vi "Main.vi"(8 "error in":errorcluster, 11 "Front Panel Emulator in":refnum<class "Front Panel Emulator.lvclass">) -> (0 "error out":errorcluster, 3 "Front Panel Emulator out":refnum<class "Front Panel Emulator.lvclass">)   [LabVIEW 2017, in "Front Panel Emulator.lvclass"]
doc: "The <b>Queued Message Handler</b> of the Worker that owns this VI."
uses:
  Front Panel Emulator.lvclass
  C:/Program Files (x86)/National Instruments/LabVIEW 2017/vi.lib/addons/_Workers/Library/Classes/Worker/Worker.lvclass
  Initialization Data.ctl
  Response Cases.ctl
  <vilib>/addons/_Workers/Library/Case Label.ctl
  Front Panel Emulator.lvclass/Front Panel Emulator.ctl
  rql_Position Changed.ctl
  rsp_Set Position.ctl
  <vilib>/addons/_Workers/Library/Classes/Message/Priority.ctl
  rql_Update LCD.ctl
  rqp_Update Temperature.ctl
  rqp_Update Humidity.ctl
  <vilib>/addons/_Workers/Library/Classes/Message Queue/Message Queue.lvclass
  <vilib>/addons/_Workers/Library/Workers.lvlib
  <vilib>/addons/_Workers/Library/Classes/Message/Message.lvclass
panel:
  in  "Position":dbl(knob) min=0.0 max=180.0 scale=0.0..180.0
  out "LCD":string
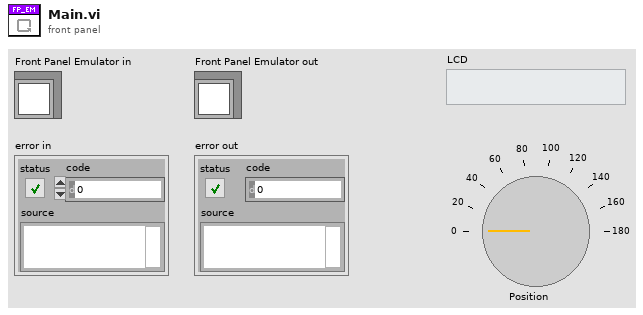
[diagram p1: front panel]
types:
  T1 = typedef "Front Panel Emulator.lvclass/Initialization Data.ctl" = cluster{"Response Cases":T2}
  T2 = typedef "Front Panel Emulator.lvclass/Response Cases.ctl" = cluster{"Set Position":T3}
  T3 = typedef "Workers.lvlib/Case Label.ctl" = string
  T4 = typedef "Front Panel Emulator.lvclass/rsp_Set Position.ctl" = cluster{"Position":dbl}
  T5 = typedef "Front Panel Emulator.lvclass/rql_Position Changed.ctl" = cluster{"Placeholder":string}
  T6 = typedef "Front Panel Emulator.lvclass/rql_Update LCD.ctl" = cluster{"Placeholder":string}
  T7 = typedef "Front Panel Emulator.lvclass/rqp_Update Temperature.ctl" = cluster{"Temperature":dbl}
  T8 = typedef "Front Panel Emulator.lvclass/rqp_Update Humidity.ctl" = cluster{"Humidity":dbl}
  T9 = typedef "Workers.lvlib/Message.lvclass/Priority.ctl" = enum16{"Low", "Normal", "High"}
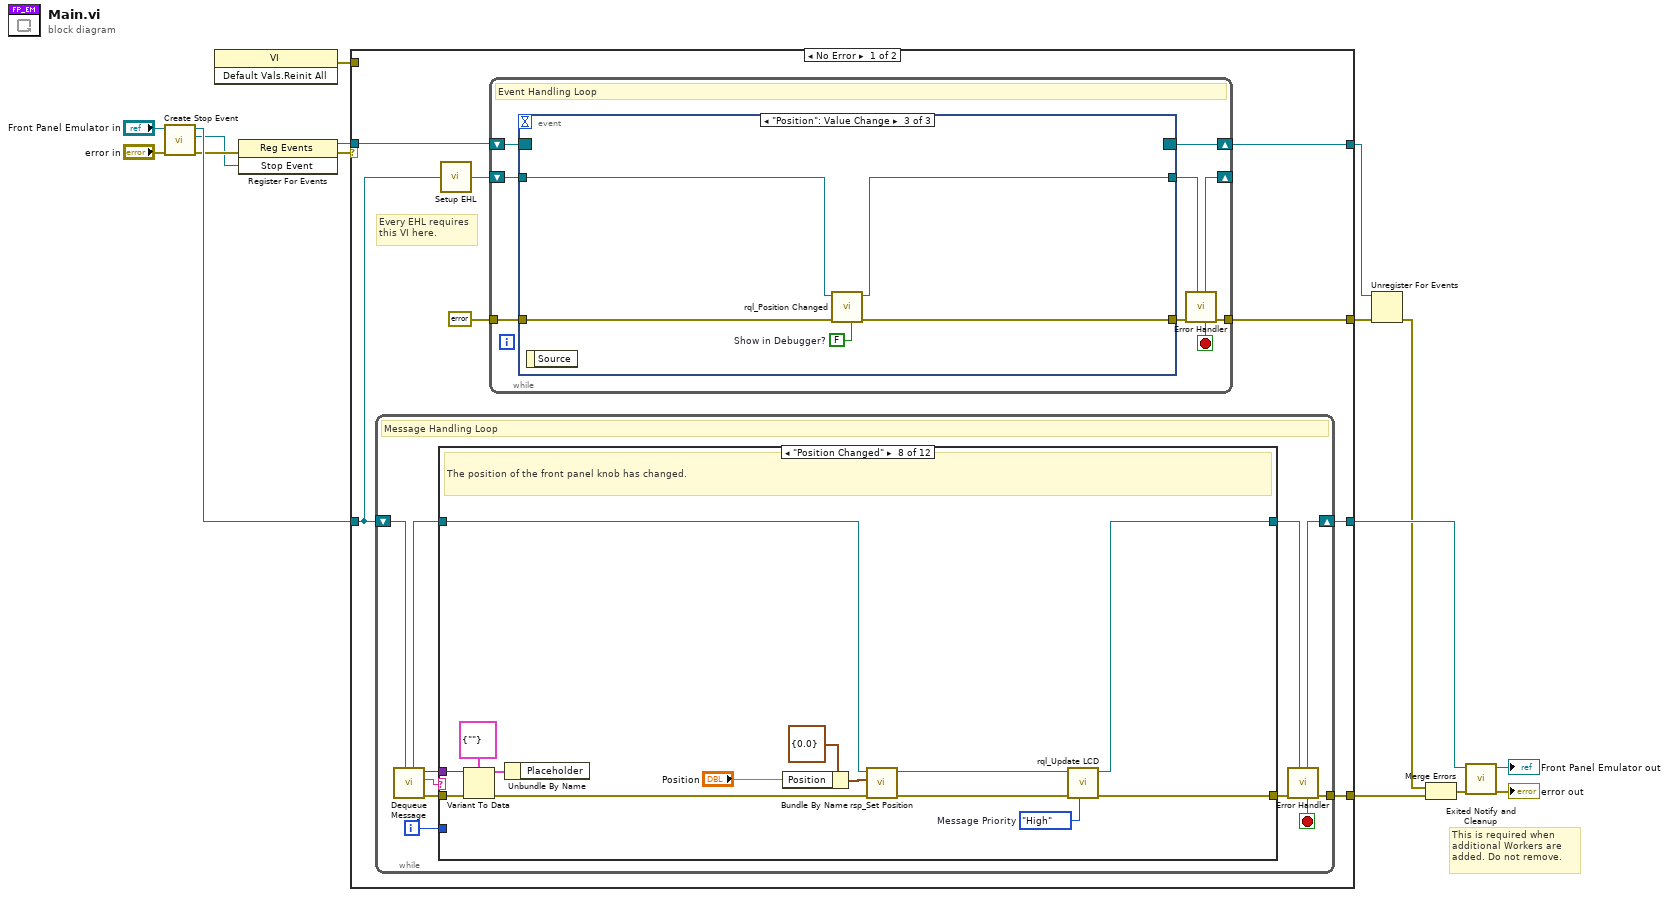
[diagram p0: block diagram]
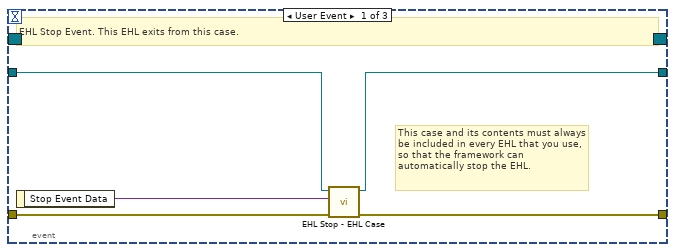
[diagram p2: hidden frame]
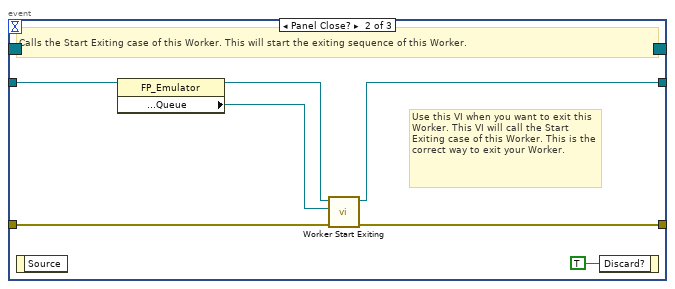
[diagram p3: hidden frame]
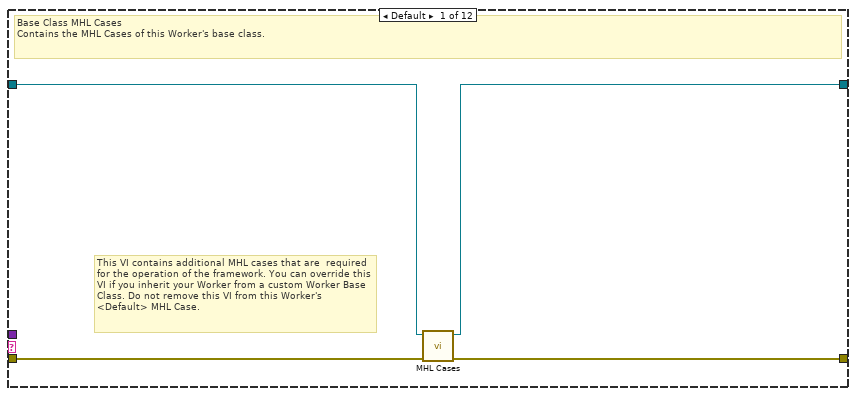
[diagram p4: hidden frame]
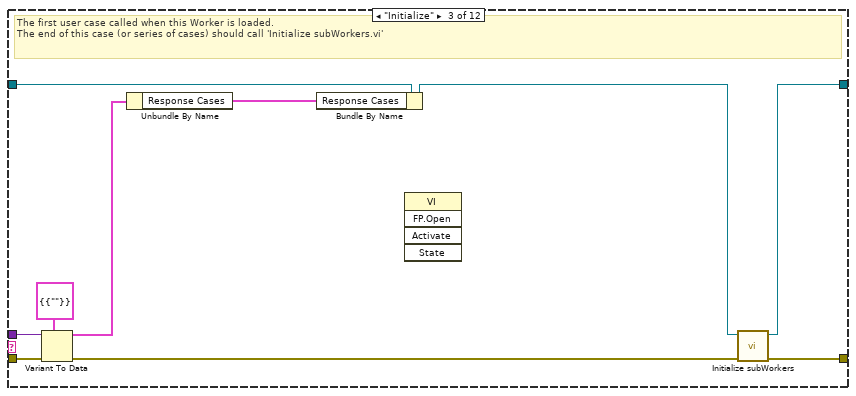
[diagram p6: hidden frame]
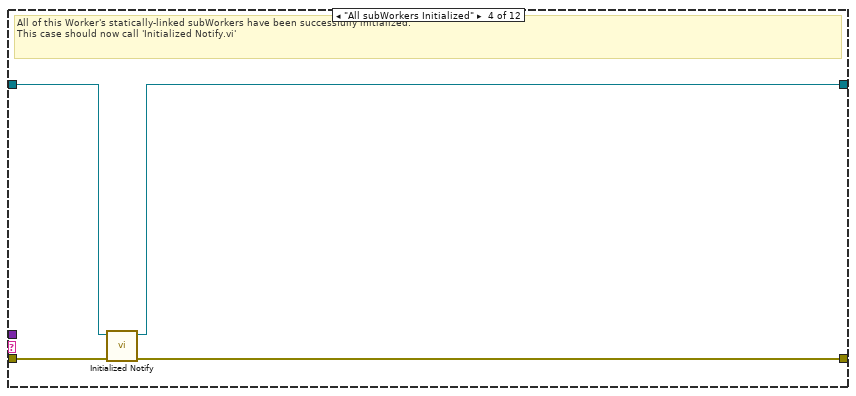
[diagram p7: hidden frame]
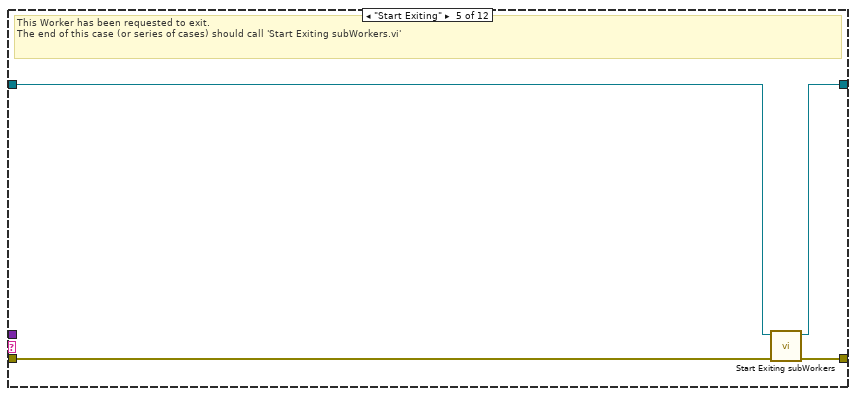
[diagram p8: hidden frame]
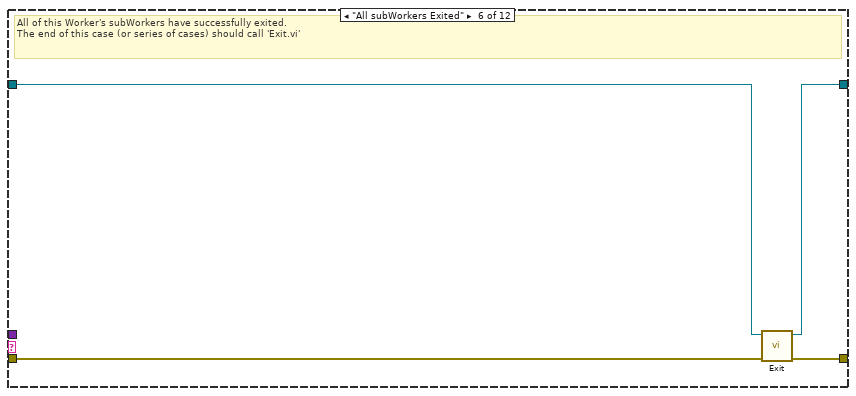
[diagram p9: hidden frame]
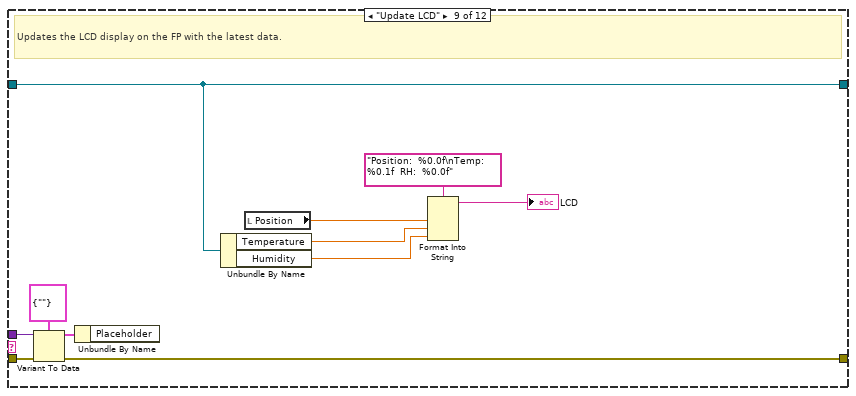
[diagram p11: hidden frame]
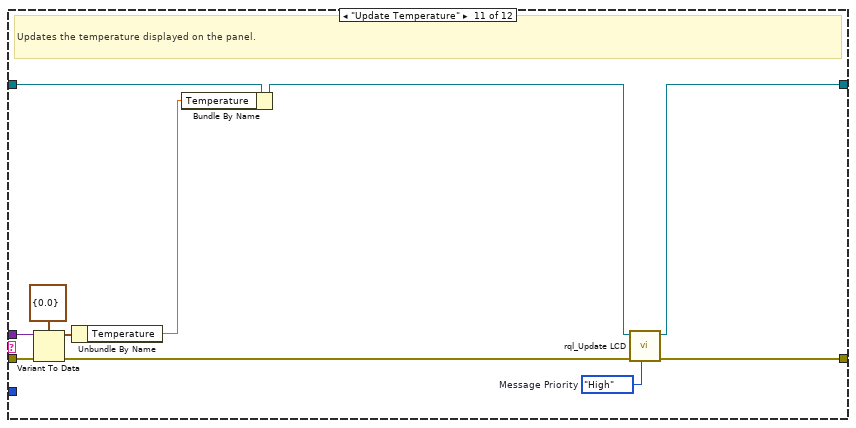
[diagram p13: hidden frame]
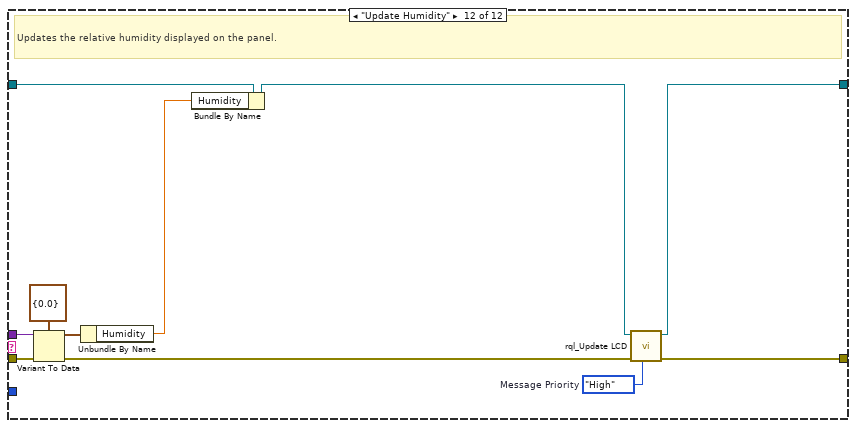
[diagram p14: hidden frame]
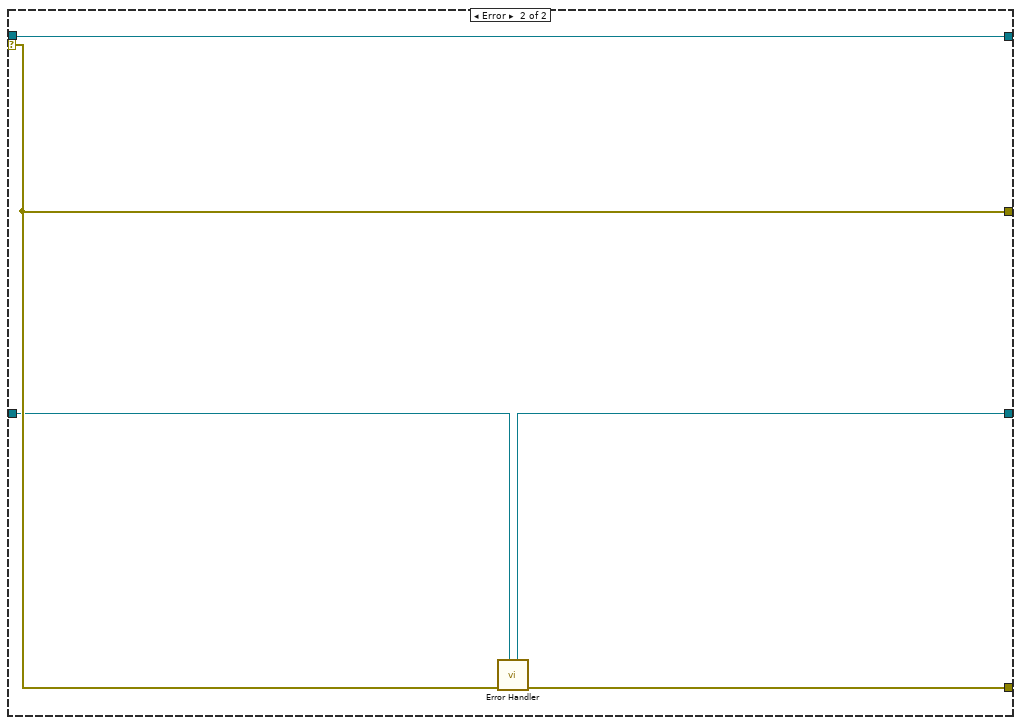
[diagram p15: hidden frame]
diagram:
  # "This is required when additional Workers are added. Do not remove."
  n1 = call-dynamic "Create Stop Event.vi"("error in"="error in", "Worker"="Front Panel Emulator in") -> ("error out"=w9:errorcluster, "Stop Event"=w8:refnum<user-event>, "Worker out"=w11:refnum<class "Front Panel Emulator.lvclass">)  [unwired: 7 in]
  n2 = invoke class="VI" method="Default Vals.Reinit All"() -> (error out=w1:errorcluster)  [unwired: 3 in, 2 out]
  n3 = register-events(error in=w9, w8) -> (reference out=w5:refnum<event-registration>, error out=w10:errorcluster)  [unwired: 1 in]
  n4 = case shown="No Error" w10 {
    tunnel: w11 -> [w22 w143]
    tunnel: [w24 w144] -> w15
    tunnel: [w23 w142] -> w16
    selector: w10 -> [_ w145]
    tunnel: w5 -> [w19 w141]
    tunnel: [w18 w141] -> w4
    tunnel: [w17 w145] -> w3
    tunnel: w1 -> [_ _]
    frame No Error {
      # "Every EHL requires\nthis VI here."
      n5 = while {
        shift-right: [w59] -> w23
        shift-left: w22 -> [w61]
        tunnel: [w60] -> w24
        i -> [w52]
        stop <- w53 stop-if-true
        # "Message Handling Loop"
        n6 = call-dynamic "Dequeue Message.vi"("Worker"=w61) -> ("error out"=w58:errorcluster, "Case out"=w54:string, "Data out"=w51:variant, "Worker out"=w56:refnum<class "Front Panel Emulator.lvclass">)  [unwired: 6 in, 1 out]
        n7 = case "Worker MHL Case Structure (DO NOT CHANGE LABEL NAME)" shown="\"Position Changed\"" w54 {
          tunnel: w58 -> [w65 w66 w75 w81 w82 w89 w91 w105 w116 w118 w128 w140]
          tunnel: [w64 w66 w77 w80 w85 w88 w91 w95 w115 w118 w123 w132] -> w57
          tunnel: w56 -> [w63 w67 w74 w79 w83 w87 w90 w99 w109 w117 w129 w134]
          tunnel: [w62 w67 w76 w78 w84 w86 w90 w93 w109 w117 w120 w133] -> w55
          tunnel: w52 -> [_ _ _ _ _ _ _ _ _ _ _ _]
          tunnel: w51 -> [_ _ w72 _ _ _ _ w102 w113 _ w125 w138]
          frame Default {
            # "This VI contains additional MHL cases that are  required for the operation of the framework. You can override this VI if you inherit your Worker from a custom Worker Base Class. Do not remove this VI from this Worker's <Default> MHL Case."
            # "Base Class MHL Cases\nContains the MHL Cases of this Worker's base class."
            n8 = call-dynamic "MHL Cases.vi"("error in"=w65, "Worker in"=w63) -> ("error out"=w64:errorcluster, "Worker out"=w62:refnum<class "Front Panel Emulator.lvclass">)  [unwired: 8 in]
          }
          frame "------------ FRAMEWORK CASES -----------" {
            # "Start of Workers Framework Cases"
          }
          frame "Initialize" {
            # "The first user case called when this Worker is loaded.\nThe end of this case (or series of cases) should call 'Initialize subWorkers.vi'"
            n9 = Variant To Data(error in=w75, type=T1 {"Response Cases"={"Set Position"=""}} ("Cluster"), Variant=w72) -> (data=w70:T1, error out=w73:errorcluster)
            n10 = Unbundle By Name(w70) -> ("Response Cases"=w69:T2)
            n11 = Bundle By Name(cluster=w74, "Response Cases"=w69) -> (w71:refnum<class "Front Panel Emulator.lvclass">)
            n12 = invoke class="VI" method="FP.Open"() -> ()  [unwired: 5 in, 5 out]
            n13 = call-dynamic "Initialize subWorkers.vi"("error in"=w73, "Worker"=w71) -> ("error out"=w77:errorcluster, "dup Worker out"=w76:refnum<class "Front Panel Emulator.lvclass">)  [unwired: 8 in]
          }
          frame "All subWorkers Initialized" {
            # "All of this Worker's statically-linked subWorkers have been successfully initialized.\nThis case should now call 'Initialized Notify.vi'"
            n14 = call-dynamic "Initialized Notify.vi"("error in"=w81, "Worker"=w79) -> ("error out"=w80:errorcluster, "dup Worker out"=w78:refnum<class "Front Panel Emulator.lvclass">)  [unwired: 8 in]
          }
          frame "Start Exiting" {
            # "This Worker has been requested to exit. \nThe end of this case (or series of cases) should call 'Start Exiting subWorkers.vi'"
            n15 = call-dynamic "Start Exiting subWorkers.vi"("error_in"=w82, "Worker"=w83) -> ("error out"=w85:errorcluster, "dup Worker out"=w84:refnum<class "Front Panel Emulator.lvclass">)  [unwired: 8 in]
          }
          frame "All subWorkers Exited" {
            # "All of this Worker's subWorkers have successfully exited. \nThe end of this case (or series of cases) should call 'Exit.vi'"
            n16 = call-dynamic "Exit.vi"("error_in"=w89, "Worker"=w87) -> ("error out"=w88:errorcluster, "dup Worker out"=w86:refnum<class "Front Panel Emulator.lvclass">)  [unwired: 8 in]
          }
          frame "------------- LOCAL API CASES -------------" {
            # "Start of Workers Local API Cases"
          }
          frame "Position Changed" {
            w92 = Priority."High"  # Message Priority
            # "The position of the front panel knob has changed."
            n17 = Variant To Data(error in=w105, type=T5 {"Placeholder"=""} ("Data"), Variant=w102) -> (data=w101:T5, error out=w104:errorcluster)
            n18 = Unbundle By Name(w101) -> ()  [unwired: 1 out]
            n19 = Bundle By Name(cluster=T4 {"Position"=0.0} ("Data in"), "Position"="Position") -> (w97:T4)
            n20 = call "rsp_Set Position.vi"("error in"=w104, "Data in"=w97, "Front Panel Emulator in"=w99) -> ("error out"=w100:errorcluster, "dup Front Panel Emulator out"=w94:refnum<class "Front Panel Emulator.lvclass">)  [unwired: 7 in]
            n21 = call "rql_Update LCD.vi"("Message Priority"=w92, "error in"=w100, "Front Panel Emulator in"=w94) -> ("error out"=w95:errorcluster, "dup Front Panel Emulator out"=w93:refnum<class "Front Panel Emulator.lvclass">)  [unwired: 7 in]
          }
          frame "Update LCD" {
            # "Updates the LCD display on the FP with the latest data."
            n22 = Variant To Data(error in=w116, type=T6 {"Placeholder"=""} ("Data"), Variant=w113) -> (data=w112:T6, error out=w115:errorcluster)
            n23 = Unbundle By Name(w112) -> ()  [unwired: 1 out]
            n24 = Unbundle By Name(w109) -> ("Temperature"=w108:dbl, "Humidity"=w107:dbl)
            n25 = local read "Position"() -> (w110:dbl)
            n26 = Format Into String(format string="Position:  %0.0f\nTemp:  %0.1f  RH:  %0.0f", w110, w108, w107) -> (resulting string=→"LCD":string)  [unwired: 2 in, 1 out]
          }
          frame "------------- PUBLIC API CASES -------------" {
            # "Start of Workers Public API Cases"
          }
          frame "Update Temperature" {
            w122 = Priority."High"  # Message Priority
            # "Updates the temperature displayed on the panel."
            n27 = Variant To Data(error in=w128, type=T7 {"Temperature"=0.0} ("Data"), Variant=w125) -> (data=w124:T7, error out=w127:errorcluster)
            n28 = Unbundle By Name(w124) -> ("Temperature"=w119:dbl)
            n29 = Bundle By Name(cluster=w129, "Temperature"=w119) -> (w121:refnum<class "Front Panel Emulator.lvclass">)
            n30 = call "rql_Update LCD.vi"("Message Priority"=w122, "error in"=w127, "Front Panel Emulator in"=w121) -> ("error out"=w123:errorcluster, "dup Front Panel Emulator out"=w120:refnum<class "Front Panel Emulator.lvclass">)  [unwired: 7 in]
          }
          frame "Update Humidity" {
            w136 = Priority."High"  # Message Priority
            # "Updates the relative humidity displayed on the panel."
            n31 = Variant To Data(error in=w140, type=T8 {"Humidity"=0.0} ("Data"), Variant=w138) -> (data=w137:T8, error out=w131:errorcluster)
            n32 = Unbundle By Name(w137) -> ("Humidity"=w130:dbl)
            n33 = Bundle By Name(cluster=w134, "Humidity"=w130) -> (w135:refnum<class "Front Panel Emulator.lvclass">)
            n34 = call "rql_Update LCD.vi"("Message Priority"=w136, "error in"=w131, "Front Panel Emulator in"=w135) -> ("error out"=w132:errorcluster, "dup Front Panel Emulator out"=w133:refnum<class "Front Panel Emulator.lvclass">)  [unwired: 7 in]
          }
        }
        n35 = call-dynamic "Error Handler.vi"("Worker"=w55, "error_in"=w57) -> ("error out"=w60:errorcluster, "Stop Loop"=w53:bool, "Worker out"=w59:refnum<class "Front Panel Emulator.lvclass">)  [unwired: 7 in]
      }
      n36 = call-dynamic "Setup EHL.vi"("Worker"=w22) -> ("Worker out"=w20:refnum<class "Front Panel Emulator.lvclass">)  [unwired: 14 in]
      n37 = while "Event Handling Loop" {
        shift-right: [w33] -> w18
        shift-left: w19 -> [w32]
        tunnel: [w28] -> w17
        tunnel: errorcluster {"status"=FALSE, "code"=0, "source"=""} ("error constant") -> [w30]
        shift-right: [w26] -> _
        shift-left: w20 -> [w31]
        stop <- w25 stop-if-true
        # "Event Handling Loop"
        n38 = event shown="[2] \"Position\": Value Change" {
          selector: w32 -> [_ _ _]
          dyn-events: [_ _ _] -> w33
          timeout: _ -> [_ _ _]
          tunnel: [w37 w44 w49] -> w29
          tunnel: w30 -> [w38 w43 w50]
          tunnel: w31 -> [w36 w42 w48]
          tunnel: [w35 w41 w47] -> w27
          event User Event {
            # "This case and its contents must always be included in every EHL that you use, so that the framework can automatically stop the EHL."
            # "EHL Stop Event. This EHL exits from this case."
            n39 = event-data() -> ("Stop Event Data"=w34:variant)  [unwired: 1 in]
            n40 = call-dynamic "EHL Stop - EHL Case.vi"("error in"=w38, "Stop Event Data"=w34, "Worker"=w36) -> ("error out"=w37:errorcluster, "Worker out"=w35:refnum<class "Front Panel Emulator.lvclass">)  [unwired: 7 in]
          }
          event Panel Close? {
            # "Use this VI when you want to exit this Worker. This VI will call the Start Exiting case of this Worker. This is the correct way to exit your Worker."
            # "Calls the Start Exiting case of this Worker. This will start the exiting sequence of this Worker."
            n41 = event-data() -> ()  [unwired: 1 in, 1 out]
            n42 = property class="FP_Emulator"(reference=w42) -> (reference out=w40:refnum<class "Front Panel Emulator.lvclass">, "Accessors:Read:Public API:Queue"=w39:refnum<class "Message Queue.lvclass">)  [unwired: 1 in, 1 out]
            n43 = call-dynamic "Worker Start Exiting.vi"("error_in"=w43, "Message Queue"=w39, "Worker"=w40) -> ("error out"=w44:errorcluster, "dup Worker out"=w41:refnum<class "Front Panel Emulator.lvclass">)  [unwired: 7 in]
            n44 = event-data("Discard?"=TRUE) -> ()  [unwired: 1 in, 1 out]
          }
          event "Position": Value Change {
            w46 = FALSE  # Show in Debugger?
            n45 = event-data() -> ()  [unwired: 1 in, 1 out]
            n46 = call "rql_Position Changed.vi"("Show in Debugger?"=w46, "error in"=w50, "Front Panel Emulator in"=w48) -> ("error out"=w49:errorcluster, "dup Front Panel Emulator out"=w47:refnum<class "Front Panel Emulator.lvclass">)  [unwired: 7 in]
          }
        }
        n47 = call-dynamic "Error Handler.vi"("Worker"=w27, "error_in"=w29) -> ("error out"=w28:errorcluster, "Stop Loop"=w25:bool, "Worker out"=w26:refnum<class "Front Panel Emulator.lvclass">)  [unwired: 7 in]
      }
    }
    frame Error {
      n48 = call-dynamic "Error Handler.vi"("Worker"=w143, "error_in"=w145) -> ("error out"=w144:errorcluster, "Worker out"=w142:refnum<class "Front Panel Emulator.lvclass">)  [unwired: 7 in, 1 out]
    }
  }
  n49 = Unregister For Events(event registration refnum=w4, error in=w3) -> (error out=w2:errorcluster)
  n50 = Merge Errors(w2, w15) -> (w12:errorcluster)
  n51 = call-dynamic "Exited Notify and Cleanup.vi"("error_in"=w12, "Worker"=w16) -> ("error out"=→"error out":errorcluster, "dup Worker out"=→"Front Panel Emulator out":refnum<class "Front Panel Emulator.lvclass">)  [unwired: 8 in]
